vi "Drive Encoder Config.vi"(0 "Left Drive Encoder Channel A":T2, 4 "Decoding Type":T1=enum."4x", 5 "Left Drive Encoder Channel B":T2, 6 "Minimum Rate":dbl=20.0, 8 "DistancePerCount":dbl=1.0, 9 "Right Drive Encoder Channel A":T2, 10 "Number Samples to Average":u8=1 min=1 max=128, 11 "Right Drive Encoder Channel B":T2, 15 "Invert Right Side":bool) -> ()   [LabVIEW 2012]
uses:
  <vilib>/Rock Robotics/SystemInterfaces/DIO/FPGA_DIOChannel.ctl
  <vilib>/Rock Robotics/WPI/Encoder/WPI_EncoderType.ctl
  <vilib>/Rock Robotics/WPI/Counter/WPI_CounterDigitalInputToDigitalSource.vi
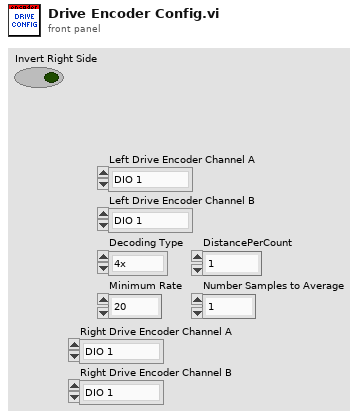
[diagram p1: front panel]
types:
  T1 = typedef "WPI_EncoderType.ctl" = enum16{"1x", "2x", "4x"}
  T2 = typedef "FPGA_DIOChannel.ctl" = enum8{"DIO 1", "DIO 2", "DIO 3", "DIO 4", "DIO 5", "DIO 6", "DIO 7", "DIO 8", "DIO 9", "DIO 10", "DIO 11", "DIO 12", "DIO 13", "DIO 14", "Invalid"}
  T3 = typedef "WPI_DigitalInputDevRef.ctl" = cluster{"DevStatus":errorcluster, "DIO Channel":T2, "Digital Module":T4}
  T4 = typedef "FPGA_TypedefDigitalModule.ctl" = enum16{"Digital Module 1", "Digital Module 2"}
  T5 = typedef "FPGA_CounterEncoderSourceConvertionLVSourceType.ctl" = cluster{"DevStatus":errorcluster, "AnalogTriggerMode?":bool, "DigitalMode":cluster{"Digital Module":T4, "DIO Channel":T6}, "AnalogTriggerMode":cluster{"AnalogTriggerIndex":T7, "OutputType":T8}}
  T6 = typedef "FPGA_DIODigitalSourceChannel.ctl" = enum8{"DIO 1", "DIO 2", "DIO 3", "DIO 4", "DIO 5", "DIO 6", "DIO 7", "DIO 8", "DIO 9", "DIO 10", "DIO 11", "DIO 12", "DIO 13", "DIO 14", "Disabled"}
  T7 = typedef "FPGA_AnalogTriggerIndex.ctl" = enum8{"Trig 0", "Trig 1", "Trig 2", "Trig 3", "Trig 4", "Trig 5", "Trig 6", "Trig 7", "Invalid"}
  T8 = typedef "FPGA_AnalogTriggerOutType.ctl" = enum16{"InWindow", "TriggerState", "Rising", "Falling"}
  T9 = typedef "WPI_EncoderDevRef.ctl" = cluster{"DevStatus":errorcluster, "EncoderIndex":T10, "CounterIndex":T11, "DistancePerCount":dbl, "Decoding Type":T1}
  T10 = typedef "FPGA_EncoderIdx.ctl" = enum8{"Enc 0", "Enc 1", "Enc 2", "Enc 3", "Invalid"}
  T11 = typedef "FPGA_CounterCtrSystemIndex.ctl" = enum8{"Ctr 0", "Ctr 1", "Ctr 2", "Ctr 3", "Ctr 4", "Ctr 5", "Ctr 6", "Ctr 7", "Invalid"}
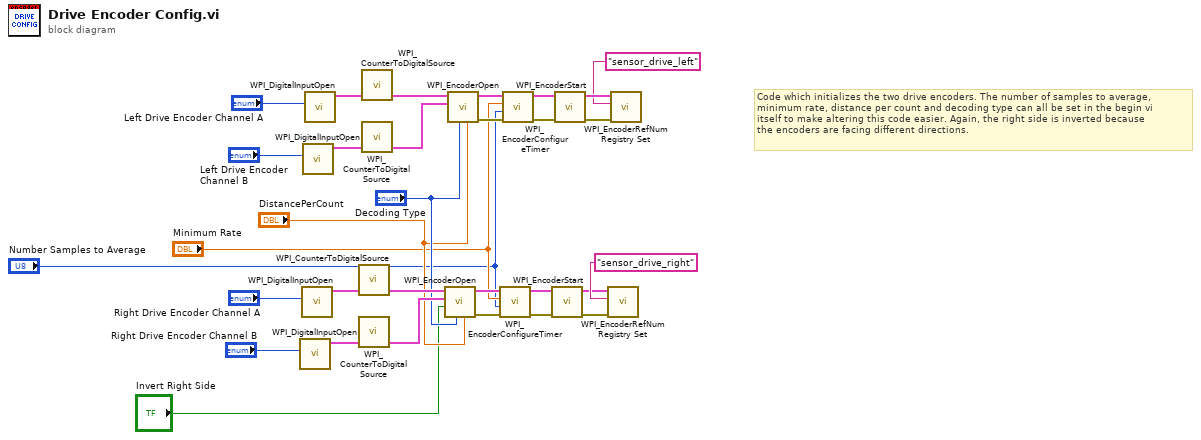
[diagram p0: block diagram]
diagram:
  # "Code which initializes the two drive encoders. The number of samples to average, \nminimum rate, distance per count and decoding type can all be set in the begin vi \nitself to make altering this code easier. Again, the right side is inverted because\nthe encoders are facing different directions."
  n1 = call <vilib>:"WPI_DigitalInputOpen.vi"("DIO Channel"="Right Drive Encoder Channel B") -> ("DigitalInputDevRef"=w7:T3)  [unwired: 9 in, 1 out]
  n2 = call <vilib>:"WPI_DigitalInputOpen.vi"("DIO Channel"="Right Drive Encoder Channel A") -> ("DigitalInputDevRef"=w6:T3)  [unwired: 9 in, 1 out]
  n3 = call <vilib>:"WPI_DigitalInputOpen.vi"("DIO Channel"="Left Drive Encoder Channel B") -> ("DigitalInputDevRef"=w30:T3)  [unwired: 9 in, 1 out]
  n4 = call <vilib>:"WPI_DigitalInputOpen.vi"("DIO Channel"="Left Drive Encoder Channel A") -> ("DigitalInputDevRef"=w31:T3)  [unwired: 9 in, 1 out]
  n5 = call-poly <vilib>:"WPI_CounterToDigitalSource.vi"("DigitalInputDevRef"=w6) -> ("Digital Source"=w10:T5)  [unwired: 6 in]
  n6 = call-poly <vilib>:"WPI_CounterToDigitalSource.vi"("DigitalInputDevRef"=w7) -> ("Digital Source"=w11:T5)  [unwired: 6 in]
  n7 = call-poly <vilib>:"WPI_CounterToDigitalSource.vi"("DigitalInputDevRef"=w31) -> ("Digital Source"=w27:T5)  [unwired: 6 in]
  n8 = call-poly <vilib>:"WPI_CounterToDigitalSource.vi"("DigitalInputDevRef"=w30) -> ("Digital Source"=w26:T5)  [unwired: 6 in]
  n9 = call <vilib>:"WPI_EncoderOpen.vi"("DistancePerCount"="DistancePerCount", "Decoding Type"="Decoding Type", "Invert Direction (False)"="Invert Right Side", "BSource"=w11, "ASource"=w10) -> ("error out"=w12:errorcluster, "EncoderDevRef"=w13:T9)  [unwired: 5 in]
  n10 = call <vilib>:"WPI_EncoderOpen.vi"("DistancePerCount"="DistancePerCount", "Decoding Type"="Decoding Type", "BSource"=w26, "ASource"=w27) -> ("error out"=w25:errorcluster, "EncoderDevRef"=w24:T9)  [unwired: 6 in]
  n11 = call <vilib>:"WPI_EncoderConfigureTimer.vi"("error in (no error)"=w12, "Number Samples to Average"="Number Samples to Average", "Minimum Rate"="Minimum Rate", "EncoderDevRef"=w13) -> ("error out"=w14:errorcluster, "EncoderDevRef"=w15:T9)  [unwired: 6 in]
  n12 = call <vilib>:"WPI_EncoderConfigureTimer.vi"("error in (no error)"=w25, "Number Samples to Average"="Number Samples to Average", "Minimum Rate"="Minimum Rate", "EncoderDevRef"=w24) -> ("error out"=w23:errorcluster, "EncoderDevRef"=w22:T9)  [unwired: 6 in]
  n13 = call <vilib>:"WPI_EncoderStart.vi"("error in (no error)"=w14, "EncoderDevRef"=w15) -> ("error out"=w16:errorcluster, "EncoderDevRef"=w17:T9)  [unwired: 8 in]
  n14 = call <vilib>:"WPI_EncoderStart.vi"("error in (no error)"=w23, "EncoderDevRef"=w22) -> ("error out"=w21:errorcluster, "EncoderDevRef"=w20:T9)  [unwired: 8 in]
  n15 = call <vilib>:"WPI_EncoderRefNum Registry Set.vi"("error in (no error)"=w16, "refnum name"="sensor_drive_right", "EncoderDevRef"=w17) -> ()  [unwired: 7 in, 2 out]
  n16 = call <vilib>:"WPI_EncoderRefNum Registry Set.vi"("error in (no error)"=w21, "refnum name"="sensor_drive_left", "EncoderDevRef"=w20) -> ()  [unwired: 7 in, 2 out]
